vi "GetWireEndpoint.vi"(4 "source":bool, 6 "terminal":refnum<class "Terminal.lvclass">, 8 "error in":errorcluster, 11 "VI Interpreter in":refnum<class "VI Interpreter.lvclass">) -> (0 "error out":errorcluster, 3 "VI Interpreter out":refnum<class "VI Interpreter.lvclass">, 5 "connection UID":i32, 7 "connection type":T1)   [LabVIEW 2014, in "Raspberry Pi Compatible Compiler for LabVIEW.lvlib" / "VI Interpreter.lvclass"]
uses:
  VI Interpreter.lvclass
  Terminal/Terminal.lvclass
  connectionType_TD.ctl
  Tunnel/Tunnel.lvclass
  FlatSequenceInnerTunnel/FlatSequenceInnerTunnel.lvclass
  FlatSequenceOuterTunnel/FlatSequenceOuterTunnel.lvclass
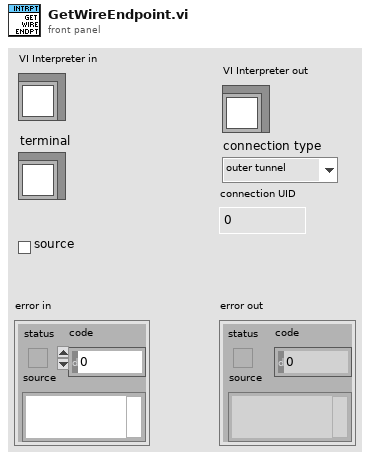
[diagram p1: front panel]
types:
  T1 = typedef "Raspberry Pi Compatible Compiler for LabVIEW.lvlib/VI Interpreter.lvclass/connectionType_TD.ctl" = enum16{"outer tunnel", "inner tunnel", "FSS outer tunnel", "FSS inner tunnel", "node"}
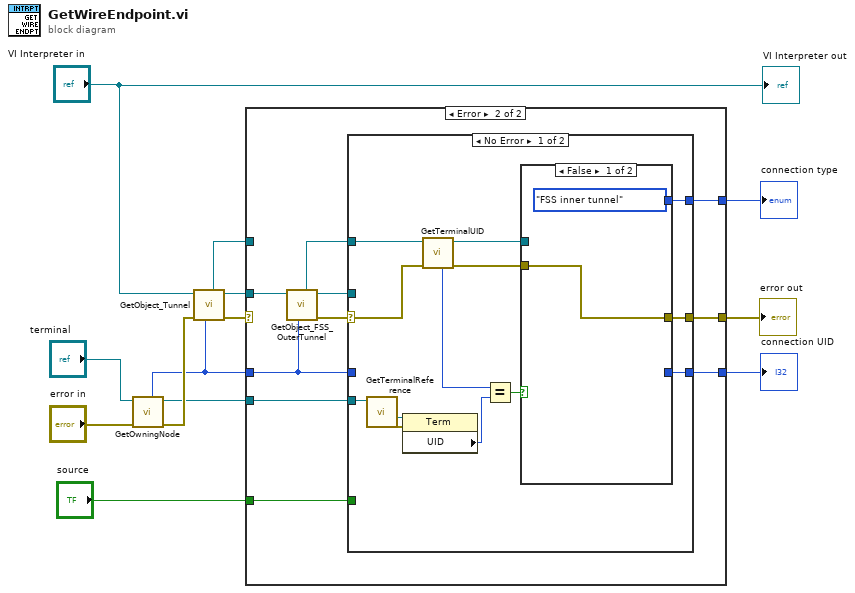
[diagram p0: block diagram]
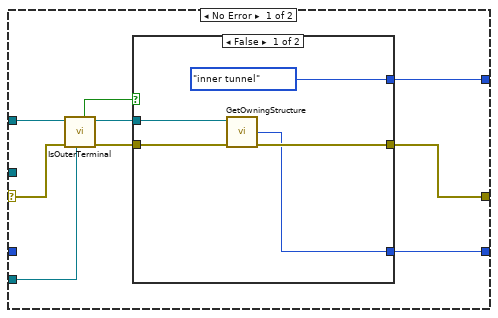
[diagram p2: hidden frame]
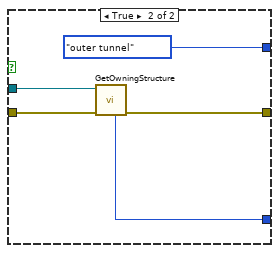
[diagram p3: hidden frame]
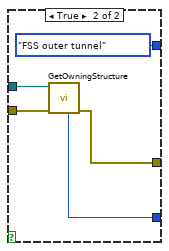
[diagram p4: hidden frame]
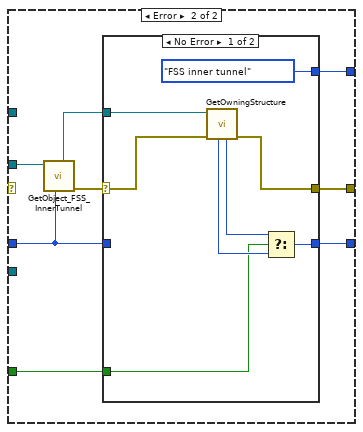
[diagram p5: hidden frame]
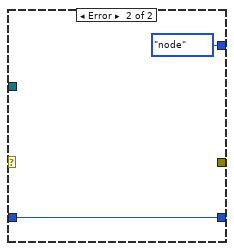
[diagram p6: hidden frame]
diagram:
  n1 = call-dynamic "GetOwningNode.vi"("error in"="error in", "Terminal in"="terminal") -> ("error out"=w9:errorcluster, "Terminal out"=w8:refnum<class "Terminal.lvclass">, "node UID"=w5:i32)  [unwired: 5 in]
  n2 = call "GetObject_Tunnel.vi"("UID"=w5, "error in"=w9, "VI Interpreter in"="VI Interpreter in") -> ("error out"=w13:errorcluster, "VI Interpreter out"=w11:refnum<class "VI Interpreter.lvclass">, "Tunnel"=w12:refnum<class "Tunnel.lvclass">)  [unwired: 3 in, 1 out]
  n3 = case shown="Error" w13 {
    selector: w13 -> [w21 _]
    tunnel: w12 -> [w22 _]
    tunnel: w11 -> [_ w42]
    tunnel: w8 -> [w20 w33]
    tunnel: [w16 w38] -> w4
    tunnel: [w15 w37] -> w6
    tunnel: w5 -> [_ w36]
    tunnel: [w14 w35] -> w2
    tunnel: "source" -> [_ w34]
    frame No Error {
      n4 = call "IsOuterTerminal.vi"("terminal"=w20, "error in"=w21, "Tunnel in"=w22) -> ("error out"=w17:errorcluster, "Tunnel out"=w18:refnum<class "Tunnel.lvclass">, "Outer"=w19:bool)  [unwired: 4 in]
      n5 = case shown="False" w19 {
        tunnel: w18 -> [w26 w31]
        tunnel: w17 -> [w25 w30]
        tunnel: [connectionType_TD."inner tunnel" connectionType_TD."outer tunnel"] -> w16
        tunnel: [w24 w28] -> w15
        tunnel: [w23 w29] -> w14
        frame False {
          n6 = call "GetOwningStructure.vi"("error in"=w25, "Tunnel in"=w26) -> ("error out"=w24:errorcluster, "UID"=w23:i32)  [unwired: 5 in, 1 out]
        }
        frame True {
          n7 = call "GetOwningStructure.vi"("error in"=w30, "Tunnel in"=w31) -> ("error out"=w28:errorcluster, "UID"=w29:i32)  [unwired: 5 in, 1 out]
        }
      }
    }
    frame Error {
      n8 = call "GetObject_FSS_OuterTunnel.vi"("UID"=w36, "VI Interpreter in"=w42) -> ("error out"=w41:errorcluster, "VI Interpreter out"=w39:refnum<class "VI Interpreter.lvclass">, "Tunnel"=w40:refnum<class "FlatSequenceOuterTunnel.lvclass">)  [unwired: 4 in, 1 out]
      n9 = case shown="No Error" w41 {
        selector: w41 -> [w50 _]
        tunnel: w40 -> [w49 _]
        tunnel: w39 -> [_ w70]
        tunnel: [w55 w67] -> w38
        tunnel: [w54 w66] -> w37
        tunnel: w36 -> [_ w65]
        tunnel: [w53 w64] -> w35
        tunnel: w34 -> [_ w63]
        tunnel: w33 -> [w48 _]
        frame No Error {
          n10 = call "GetTerminalReference.vi"("Terminal in"=w48) -> ("error out"=w47:errorcluster, "reference"=w46:refnum<vi>)  [unwired: 8 in, 1 out]
          n11 = property class="Term"(reference=w46, error in=w47) -> ("UID"=w45:i32)  [unwired: 2 out]
          n12 = call "GetTerminalUID.vi"("error in"=w50, "Tunnel in"=w49) -> ("error out"=w51:errorcluster, "Tunnel out"=w52:refnum<class "FlatSequenceOuterTunnel.lvclass">, "outside terminal UID"=w43:i32)  [unwired: 4 in, 1 out]
          n13 = Equal?(x=w43, y=w45) -> (x = y?=w44:bool)
          n14 = case shown="False" w44 {
            tunnel: [connectionType_TD."FSS inner tunnel" connectionType_TD."FSS outer tunnel"] -> w55
            tunnel: [w56 w61] -> w54
            tunnel: [_ w60] -> w53
            tunnel: w52 -> [_ w59]
            tunnel: w51 -> [w56 w58]
            frame False {
            }
            frame True {
              n15 = call "GetOwningStructure.vi"("error in"=w58, "Tunnel in"=w59) -> ("error out"=w61:errorcluster, "UID"=w60:i32)  [unwired: 5 in, 1 out]
            }
          }
        }
        frame Error {
          n16 = call "GetObject_FSS_InnerTunnel.vi"("UID"=w65, "VI Interpreter in"=w70) -> ("error out"=w69:errorcluster, "Tunnel"=w68:refnum<class "FlatSequenceInnerTunnel.lvclass">)  [unwired: 4 in, 2 out]
          n17 = case shown="No Error" w69 {
            selector: w69 -> [w76 _]
            tunnel: w68 -> [w77 _]
            tunnel: [connectionType_TD."FSS inner tunnel" ("Enum") connectionType_TD."node" ("Enum")] -> w67
            tunnel: [w75 _] -> w66
            tunnel: w65 -> [_ w79]
            tunnel: [w71 w79] -> w64
            tunnel: w63 -> [w72 _]
            frame No Error {
              n18 = call "GetOwningStructure.vi"("error in"=w76, "Tunnel in"=w77) -> ("error out"=w75:errorcluster, "right frame"=w74:i32, "left frame"=w73:i32)  [unwired: 4 in, 1 out]
              n19 = Select(t=w74, s=w72, f=w73) -> (s? t:f=w71:i32)
            }
            frame Error {
            }
          }
        }
      }
    }
  }
  "error out" <- w6
  "connection type" <- w4
  "connection UID" <- w2
  "VI Interpreter out" <- "VI Interpreter in"
